vi "DestroyModuleBroadcasts.vi"(8 "error in (no error)":errorcluster, 11 "TesterModule in":refnum<class "TesterModule.lvclass">) -> (0 "error out":errorcluster, 3 "TesterModule out":refnum<class "TesterModule.lvclass">)   [LabVIEW 2024, in "TesterModule.lvclass"]
uses:
  TesterModule.lvclass
  TesterModule.lvclass/TesterModule.ctl
  JQMHCore/Module/JQMHModule.lvclass
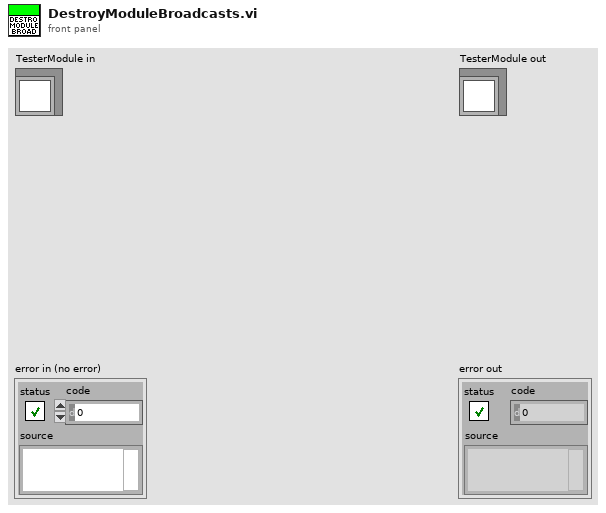
[diagram p1: front panel]
types:
  T1 = typedef "TesterModule.lvclass/Broadcasts.ctl" = cluster{"Stopped":refnum<user-event>}
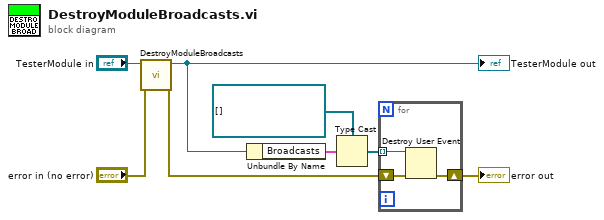
[diagram p0: block diagram]
diagram:
  n1 = call-parent "DestroyModuleBroadcasts.vi"("error in (no error)"="error in (no error)", "JQMHModule in"="TesterModule in") -> ("error out"=w1:errorcluster, "JQMHModule out"=w3:refnum<class "TesterModule.lvclass">)  [unwired: 8 in]
  "TesterModule out" <- w3
  n2 = Unbundle By Name(w3) -> ("Broadcasts"=w7:T1)
  n3 = Type Cast(type=refnum<user-event>[] [] ("NewControl5"), x=w7) -> (*(type *) &x=w6:refnum<user-event>[])
  n4 = for {
    tunnel: w6 -> [w11] mode=indexing
    shift-right: [w9] -> w5
    shift-left: w1 -> [w10]
    n5 = Destroy User Event(user event=w11, error in=w10) -> (error out=w9:errorcluster)
  }
  "error out" <- w5
